vi "FlatToRichcif_pluginloader_DiscoverCommand.vi"(5 "OutputClusterType":T1, 11 "InputCluster":T2) -> (3 "OutputCluster":T1)   [LabVIEW 2021, in "CIF_PluginLoader_client.lvlib"]
uses:
  cif_pluginloader_DiscoverCommand_Flat.ctl
  cif_pluginloader_DiscoverCommand.ctl
  CIF_PluginLoader_client.lvlib
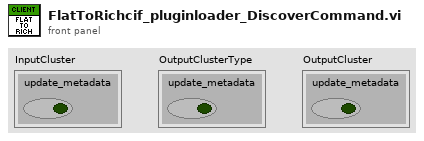
[diagram p1: front panel]
types:
  T1 = typedef "CIF_PluginLoader_client.lvlib/cif_pluginloader_DiscoverCommand.ctl" = cluster{"update_metadata":bool}
  T2 = typedef "CIF_PluginLoader_client.lvlib/cif_pluginloader_DiscoverCommand_Flat.ctl" = cluster{"update_metadata":bool}
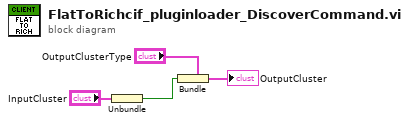
[diagram p0: block diagram]
diagram:
  n1 = Unbundle "Unbundle"("InputCluster") -> ("update_metadata"=w1:bool)
  n2 = Bundle "Bundle"(cluster="OutputClusterType", "update_metadata"=w1) -> (→"OutputCluster":T1)
